vi "COMI US Start Ex.vi"(7 "nBufSizeGain":u32, 9 "nFrameSize":u32, 10 "dwScanFreq":u32, 11 "hDevice":u32) -> (2 "function return":i32, 3 "hDevice out":u32)   [LabVIEW 2017, in "Comidll.lvlib"]
doc: "long (COMI_US_StartEx) (HANDLE hDevice, unsigned int dwScanFreq, unsigned int nFrameSize, unsigned int nBufSizeGain);"
uses:
  <userlib>/Comidll/Comidll.lvlib
  <userlib>/Comidll/Comidll.dll
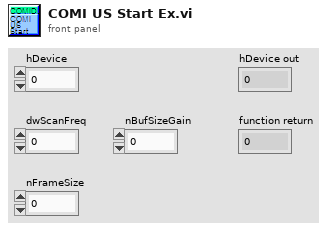
[diagram p1: front panel]
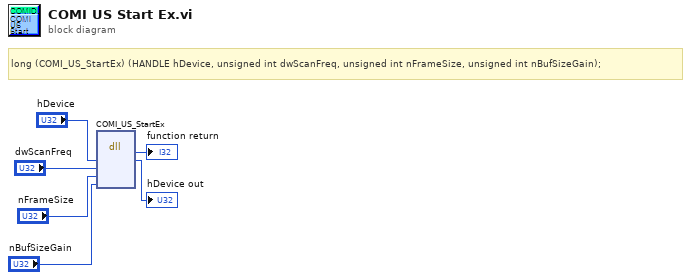
[diagram p0: block diagram]
diagram:
  # "long\t(COMI_US_StartEx) (HANDLE hDevice, unsigned int dwScanFreq, unsigned int nFrameSize, unsigned int nBufSizeGain);"
  n1 = dll-call lib="C:/Program Files/National Instruments/LabVIEW 2017/user.lib/Comidll/Comidll.*" fn="COMI_US_StartEx"("hDevice"="hDevice", "dwScanFreq"="dwScanFreq", "nFrameSize"="nFrameSize", "nBufSizeGain"="nBufSizeGain") -> (→"function return":i32, "hDevice"=→"hDevice out":u32)  [unwired: 6 in, 2 out]
